vi "Get Joystick Axis Translation.vi"(8 "error in (no error)":errorcluster, 9 "Joystick Device Number":string, 10 "Joystick Axis Number (1)":u8=1 min=1, 11 "VISA resource name":refnum<visa-resource-name>) -> (0 "error out":errorcluster, 1 "Target Speed Profile":u16(ring)=1 items=["linear"=1, "squared"=2, "cubed"=3], 2 "Maximum Speed":i32, 3 "VISA resource name out":refnum<visa-resource-name>, 4 "Resolution":i32, 5 "Joystick Axis Inverted":bool)   [LabVIEW 2015, in "Zaber A Series.lvlib"]
doc: "Use this VI to determine how movement of one joystick axis is translated into movement commands for the targeted motion device axis.\n\nInputs are the device number of the joystick to query, and the joystick axis number to check - 1 is the X axis, 2 is Y and 3 is the rotation of the knob on the end of the joystick.\n\nOutputs:\n\nMaximum speed - the highest speed that the joystick will send to the targeted axis.\n\nTarget Speed Profile - the type of curve used to map joystick positons to velocities.\n\nJoystick Axis Inverted - true if positive joystick deflection will produce negative velocities.\n\nResolution - how many discrete steps of velocity the joystick axis has.\n\nThis VI expects the serial port to have already been initialized."
uses:
  Zaber A Series.lvlib
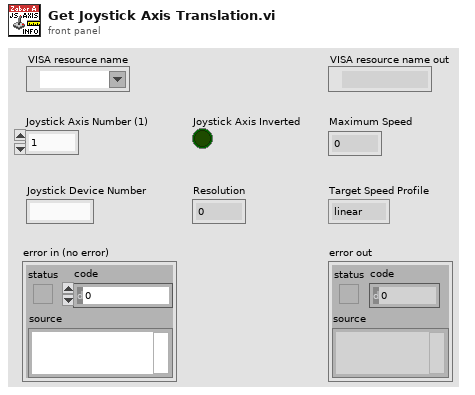
[diagram p1: front panel]
types:
  T1 = cluster{"Device":string, "Axis":string, "Reply Flag":string, "Status":string, "Warning Flags":string, "Data":string}
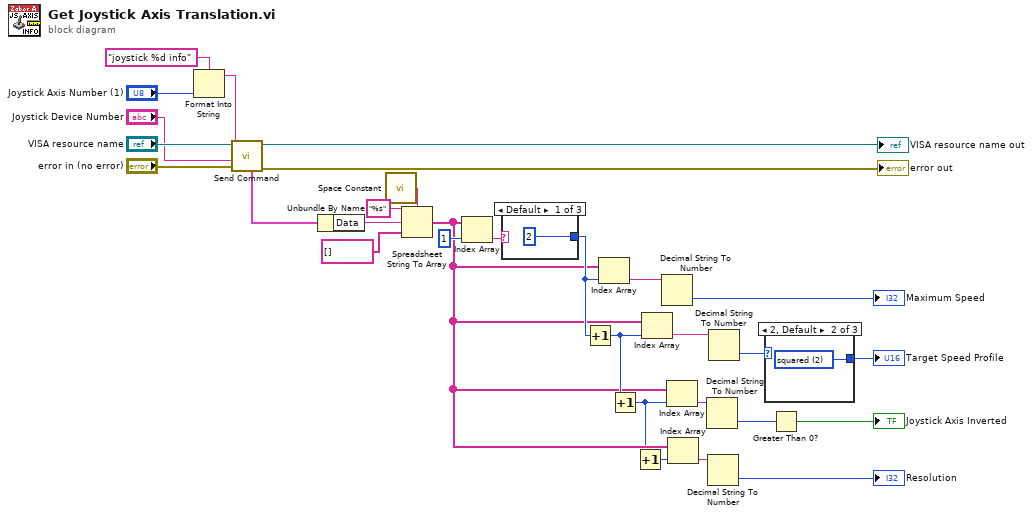
[diagram p0: block diagram]
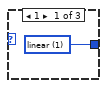
[diagram p2: hidden frame]
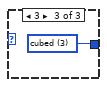
[diagram p3: hidden frame]
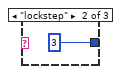
[diagram p4: hidden frame]
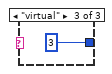
[diagram p5: hidden frame]
diagram:
  n1 = Format Into String(format string="joystick %d info", "Joystick Axis Number (1)") -> (resulting string=w6:string)  [unwired: 2 in, 1 out]
  n2 = call "Send Command.vi"("error in (no error)"="error in (no error)", "Device and Axis"="Joystick Device Number", "Command"=w6, "VISA resource name"="VISA resource name") -> ("error out"=→"error out":errorcluster, "VISA resource name out"=→"VISA resource name out":refnum<visa-resource-name>, "First Response Bundle"=w1:T1)  [unwired: 2 in, 3 out]
  n3 = Unbundle By Name(w1) -> ("Data"=w27:string)
  n4 = call <vilib>:"Space Constant.vi"() -> ("String"=w25:string)
  n5 = Spreadsheet String To Array(delimiter (Tab)=w25, format string="%s", spreadsheet string=w27, array type (2D Dbl)=string[] []) -> (array=w10:string[])
  n6 = Index Array(array=w10, index=1) -> (element=w22:string)
  n7 = case shown="Default" w22 {
    tunnel: [2 3 3] -> w15
    frame Default {
    }
    frame "lockstep" {
    }
    frame "virtual" {
    }
  }
  n8 = Increment(x=w15) -> (x+1=w14:i32)
  n9 = Index Array(array=w10, index=w15) -> (element=w21:string)
  n10 = Increment(x=w14) -> (x+1=w9:i32)
  n11 = Increment(x=w9) -> (x+1=w12:i32)
  n12 = Index Array(array=w10, index=w14) -> (element=w16:string)
  n13 = Decimal String To Number(string=w21) -> (number=→"Maximum Speed":i32)  [unwired: 2 in, 1 out]
  n14 = Index Array(array=w10, index=w9) -> (element=w19:string)
  n15 = Index Array(array=w10, index=w12) -> (element=w11:string)
  n16 = Decimal String To Number(string=w19) -> (number=w18:i32)  [unwired: 2 in, 1 out]
  n17 = Decimal String To Number(string=w11) -> (number=→"Resolution":i32)  [unwired: 2 in, 1 out]
  n18 = Decimal String To Number(string=w16) -> (number=w13:i32)  [unwired: 2 in, 1 out]
  n19 = case shown="2, Default" w13 {
    tunnel: [w34 w35 w36] -> w2
    frame 1 {
      w34 = u16 1 items=["linear"=1, "squared"=2, "cubed"=3]
    }
    frame 2, Default {
      w35 = u16 2 items=["linear"=1, "squared"=2, "cubed"=3]
    }
    frame 3 {
      w36 = u16 3 items=["linear"=1, "squared"=2, "cubed"=3]
    }
  }
  "Target Speed Profile" <- w2
  n20 = Greater Than 0?(x=w18) -> (x > 0?=→"Joystick Axis Inverted":bool)
